vi "calcStiffness.vi"(8 "error in (no error)":errorcluster, 11 "Model in":refnum<class "Model.lvclass">) -> (0 "error out":errorcluster, 3 "Model out":refnum<class "Model.lvclass">)   [LabVIEW 2015]
uses:
  ApplicationElements/StiffnessMonitor/StiffnessMonitor.lvclass
  Typedefs/StiffnessData.ctl
  Typedefs/M1M3SSSTypedefs.lvlib
  UserEvents/UserEvents.lvclass
  <userlib>/Common/Devices/DistanceGauge/DistanceGauge/DistanceGauge.lvclass
  <userlib>/Common/Devices/ForceSensorCalculator/ForceSensorCalculator/ForceSensorCalculator.lvclass
  ApplicationElements/Log/StiffnessLog/StiffnessLog.lvclass
  Model.lvclass
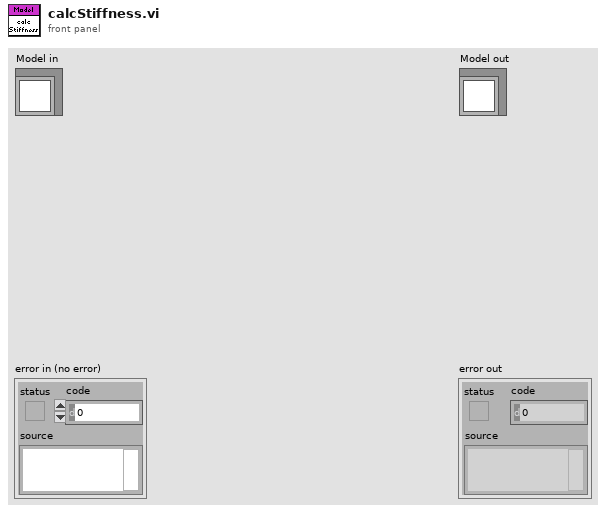
[diagram p1: front panel]
types:
  T1 = typedef "M1M3SSSTypedefs.lvlib/StiffnessData.ctl" = cluster{"Constrained Displacement":dbl[unit], "Stiffness":dbl[unit]}
  T2 = typedef "M1M3SSSTypedefs.lvlib/PubDataEvents.ctl" = cluster{"State":refnum<user-event>, "ErrorCode":refnum<user-event>, "OutputData":refnum<user-event>, "InputData":refnum<user-event>, "ControllerData":refnum<user-event>, "TestStatus":refnum<user-event>, "LogPath":refnum<user-event>, "StiffnessData":refnum<user-event>, "PreconditioningCycle":refnum<user-event>}
  T3 = typedef "DistanceGauge.lvlib/Distance Data.ctl" = cluster{"Distance Measured":dbl[unit]}
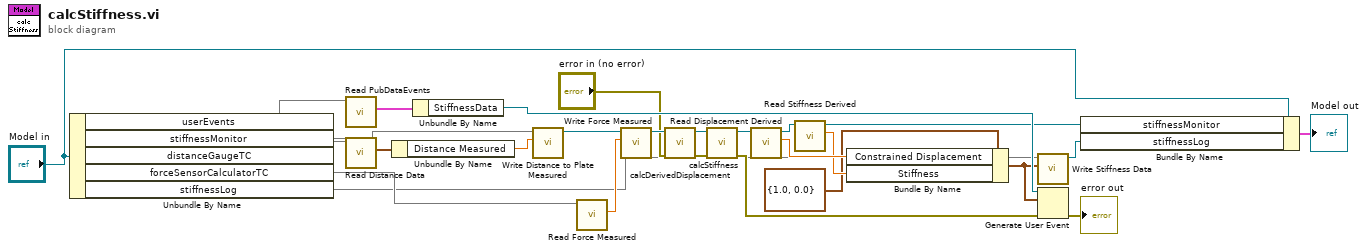
[diagram p0: block diagram]
diagram:
  n1 = Unbundle By Name("Model in") -> ("userEvents"=w18, "stiffnessMonitor"=w12, "distanceGaugeTC"=w15, "forceSensorCalculatorTC"=w14, "stiffnessLog"=w7)
  n2 = call "Read PubDataEvents.vi"("UserEvents in"=w18) -> ("PubDataEvents"=w20:T2)  [unwired: 9 in, 1 out]
  n3 = call <userlib>:"Read Distance Data.vi"("DistanceGauge in"=w15) -> ("Distance Data"=w16:T3)  [unwired: 9 in, 1 out]
  n4 = Unbundle By Name(w16) -> ("Distance Measured"=w17:dbl[unit])
  n5 = Unbundle By Name(w20) -> ("StiffnessData"=w19:refnum<user-event>)
  n6 = call "Write Distance to Plate Measured.vi"("Distance to Plate Measured"=w17, "StiffnessMonitor in"=w12) -> ("StiffnessMonitor out"=w1:refnum<class "StiffnessMonitor.lvclass">)  [unwired: 9 in]
  n7 = call <userlib>:"Read Force Measured.vi"("ForceSensor in"=w14) -> ("Force Demand"=w13:dbl[unit])  [unwired: 9 in, 1 out]
  n8 = call "Write Force Measured.vi"("Force Measured"=w13, "StiffnessMonitor in"=w1) -> ("StiffnessMonitor out"=w27:refnum<class "StiffnessMonitor.lvclass">)  [unwired: 9 in]
  n9 = call "calcDerivedDisplacement.vi"("error in (no error)"="error in (no error)", "StiffnessMonitor in"=w27) -> ("error out"=w10:errorcluster, "StiffnessMonitor out"=w26:refnum<class "StiffnessMonitor.lvclass">)  [unwired: 8 in]
  n10 = call "calcStiffness.vi"("error in (no error)"=w10, "StiffnessMonitor in"=w26) -> ("error out"=w9:errorcluster, "StiffnessMonitor out"=w25:refnum<class "StiffnessMonitor.lvclass">)  [unwired: 8 in]
  n11 = call "Read Displacement Derived.vi"("StiffnessMonitor in"=w25) -> ("Displacement Derived"=w23:dbl[unit], "StiffnessMonitor out"=w24:refnum<class "StiffnessMonitor.lvclass">)  [unwired: 9 in]
  n12 = call "Read Stiffness Derived.vi"("StiffnessMonitor in"=w24) -> ("Stiffness Derived"=w22:dbl[unit], "StiffnessMonitor out"=w3:refnum<class "StiffnessMonitor.lvclass">)  [unwired: 9 in]
  n13 = Bundle By Name(cluster=T1 {"Constrained Displacement"=1.0, "Stiffness"=0.0} ("event data"), "Constrained Displacement"=w23, "Stiffness"=w22) -> (w2:T1)
  n14 = call "Write Stiffness Data.vi"("Stiffness Data"=w2, "StiffnessLog in"=w7) -> ("StiffnessLog out"=w4:refnum<class "StiffnessLog.lvclass">)  [unwired: 9 in]
  n15 = Generate User Event(user event=w19, event data cluster=w2, error in=w9) -> (error out=→"error out":errorcluster)  [unwired: 1 in, 1 out]
  n16 = Bundle By Name(cluster="Model in", "stiffnessMonitor"=w3, "stiffnessLog"=w4) -> (→"Model out":cluster{})
